vi "Memory.Pointer.Parameter Check.Size.Base2.vi"(5 "power of 2":i16, 7 "source vi name":string, 8 "error in (no error)":errorcluster, 9 "transfer count":u64 format="%08x bytes", 10 "buffer element count":u64 format="%08x bytes", 11 "Pointer in":refnum<class "Memory.Pointer.lvclass">) -> (0 "error out":errorcluster, 1 "transfer count out":u64 format="%08x bytes", 2 "buffer element count out":u64 format="%08x bytes", 3 "Pointer out":refnum<class "Memory.Pointer.lvclass">)   [LabVIEW 2016, in "Memory Manager.lvlib" / "Memory.Pointer.lvclass"]
uses:
  Memory.Pointer.lvclass
  Memory.Pointer.lvclass/Memory.Pointer.ctl
  Memory.Pointer.Errors.Buffer Underflow.vi
  Memory.Pointer.Errors.Create Error.vi
  Submodules/Static Error Handling/Source/Library/VIs/Static Error Handling.Source Buffer.Write.String.vi
  Submodules/Static Error Handling/Source/Library/VIs/Static Error Handling.Source Buffer.Write.Numeric.Scalar.Base10.vi
  Submodules/Static Error Handling/Source/Library/VIs/Static Error Handling.Source Buffer.Write.Numeric.Scalar.Base10 (U64).vi
  Memory.Pointer.Errors.Out of Bounds.vi
  Accessors/Get Size.vi
  Submodules/Static Error Handling/Source/Library/VIs/Static Error Handling.Error Cluster Constant.vi
  Submodules/Static Error Handling/Source/Library/VIs/Static Error Handling.Error Cluster Constant (256B).vi
  Submodules/Static Error Handling/Source/Library/VIs/Static Error Handling.Parameters.Status.Set.vi
  Submodules/Static Error Handling/Source/Library/VIs/Static Error Handling.Parameters.Code.Set.vi
  Submodules/Static Error Handling/Source/Library/VIs/Static Error Handling.Parameters.VI Source.Set.vi
  Constants/Memory.Constants.vi
  Constants/Memory.Constants.Library Name.vi
  Memory.Pointer.Errors.Get Info.vi
  Memory.Pointer.Errors.Write Pointer Size.vi
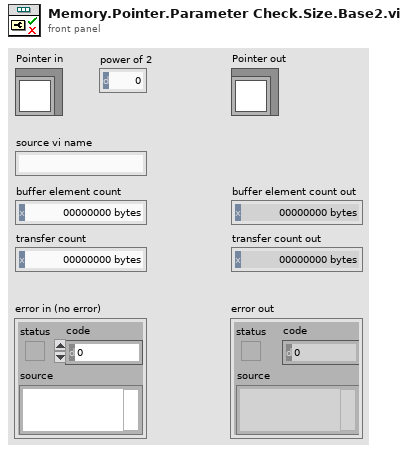
[diagram p1: front panel]
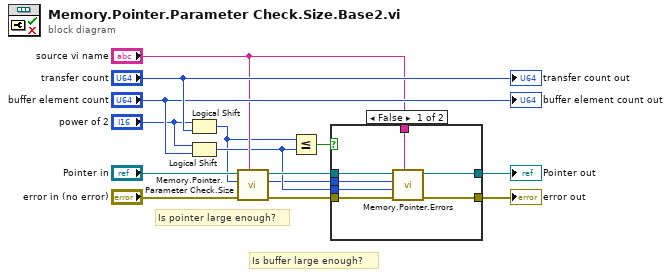
[diagram p0: block diagram]
diagram:
  # "Is buffer large enough?"
  # "Is pointer large enough?"
  n1 = Logical Shift(y="power of 2", x="transfer count") -> (x << y=w4:u64)
  n2 = Logical Shift(y="power of 2", x="buffer element count") -> (x << y=w5:u64)
  n3 = call "Memory.Pointer.Parameter Check.Size.vi"("source vi name"="source vi name", "error in (no error)"="error in (no error)", "required size"=w4, "Pointer in"="Pointer in") -> ("error out"=w6:errorcluster, "required size out"=w2:u64, "Pointer out"=w7:refnum<class "Memory.Pointer.lvclass">)  [unwired: 5 in]
  n4 = Less Or Equal?(x=w4, y=w5) -> (x <= y?=w1:bool)
  n5 = case shown="False" w1 {
    tunnel: w7 -> [w21 w22]
    tunnel: w6 -> [w19 w23]
    tunnel: [w18 w23] -> w14
    tunnel: [w20 w22] -> w13
    tunnel: "source vi name" -> [w17 _]
    tunnel: w5 -> [w16 _]
    tunnel: w2 -> [w15 _]
    frame False {
      n6 = call-poly "Memory.Pointer.Errors.vi"("source vi name"=w17, "error in (no error)"=w19, "actual buffer size"=w16, "required buffer size"=w15, "pointer in"=w21) -> ("error out"=w18:errorcluster, "pointer out"=w20:refnum<class "Memory.Pointer.lvclass">)  [unwired: 5 in]
    }
    frame True {
    }
  }
  "error out" <- w14
  "Pointer out" <- w13
  "transfer count out" <- "transfer count"
  "buffer element count out" <- "buffer element count"
